vi "Process_old.vi"(8 "error in (no error)":errorcluster, 10 "DAQ Class.lvclass":refnum<class "DAQ Class.lvclass">, 11 "Intensity Processing in":refnum<class "Intensity Processing.lvclass">) -> (0 "error out":errorcluster, 3 "Intensity Processing out":refnum<class "Intensity Processing.lvclass">)   [LabVIEW 2014]
uses:
  <vilib>/Analysis/NI_AALPro.lvlib
  DAQ/DAQ Control Functional Global States.ctl
  <vilib>/Analysis/4window.llb/Hanning Window (DBL).vi
  <vilib>/Analysis/2dsp.llb/Real FFT.vi
  DAQ/DAQ Class.lvclass
  Processing.lvclass
  Intensity Processing.lvclass
panel:
  out "Log?":bool=TRUE
  out "Intensity Graph":sgl[][](graph)
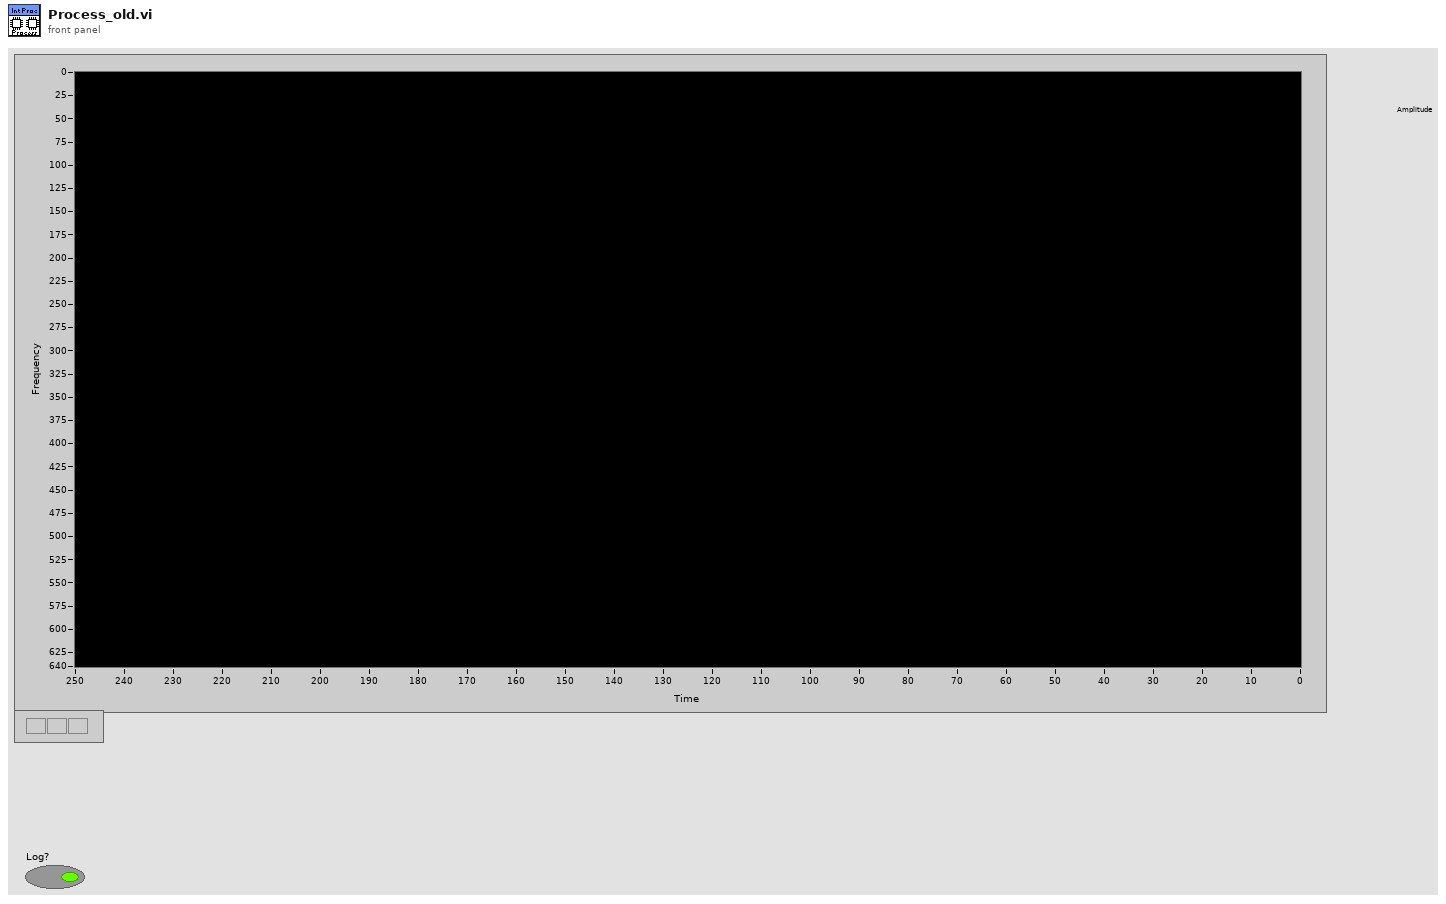
[diagram p1: front panel]
types:
  T1 = typedef "DAQ Class.lvclass/DAQ Parameters.ctl" = cluster{"Points Per A-Scan":u32, "A-Scans Per B-Scan":u32, "Number of B-Scans":u32, "A-Scans Per Transfer":u32, "Trigger Voltage":sgl, "Trigger Source":T2, "Trigger Slope":T3, "Channel":T4, "Clock":T5, "Bits per Sample":dbl, "Range":dbl}
  T2 = typedef "DAQ Class.lvclass/Trigger Source.ctl" = enum16{"External", "Channel A", "Channel B"}
  T3 = typedef "DAQ Class.lvclass/Trigger Slope.ctl" = enum16{"Rising", "Falling"}
  T4 = typedef "OCT DAQ Channel Data Type.ctl" = enum16{"Channel 1", "Channel 2", "Channel 1 and 2"}
  T5 = typedef "DAQ Class.lvclass/Clock Control.ctl" = enum16{"Internal Clock", "External Clock"}
  T6 = enum16{"open", "replace", "create", "open or create", "replace or create", "replace or create with confirmation"}
  T7 = typedef "DAQ Control Functional Global States.ctl" = enum16{"Status", "Set Processing Finished", "Reset", "Clear", "Set DAQ Finished"}
  T8 = typedef "LVCursorListTypeDef.ctl" = cluster{"Name":string, "Color":u32, "Style":u8, "Point Style":u8, "Name Visible":bool, "Allow Drag":bool, "Cursor Mode":u32, "Plot":i32, "Index":i32, "Position":cluster{"X":dbl, "Y":dbl}, "X Scale":u32, "Y Scale":u32, "Watch Plots":i32[], "Watch All Plots":bool, "Plot Area":i32, "Label Offset":cluster{"X":dbl, "Y":dbl}}[]
  T9 = cluster{"Name":string, "Color":u32, "Style":u8, "Point Style":u8, "Name Visible":bool, "Allow Drag":bool, "Cursor Mode":u32, "Plot":i32, "Index":i32, "Position":cluster{"X":dbl, "Y":dbl}, "X Scale":u32, "Y Scale":u32, "Watch Plots":i32[], "Watch All Plots":bool, "Plot Area":i32, "Label Offset":cluster{"X":dbl, "Y":dbl}}
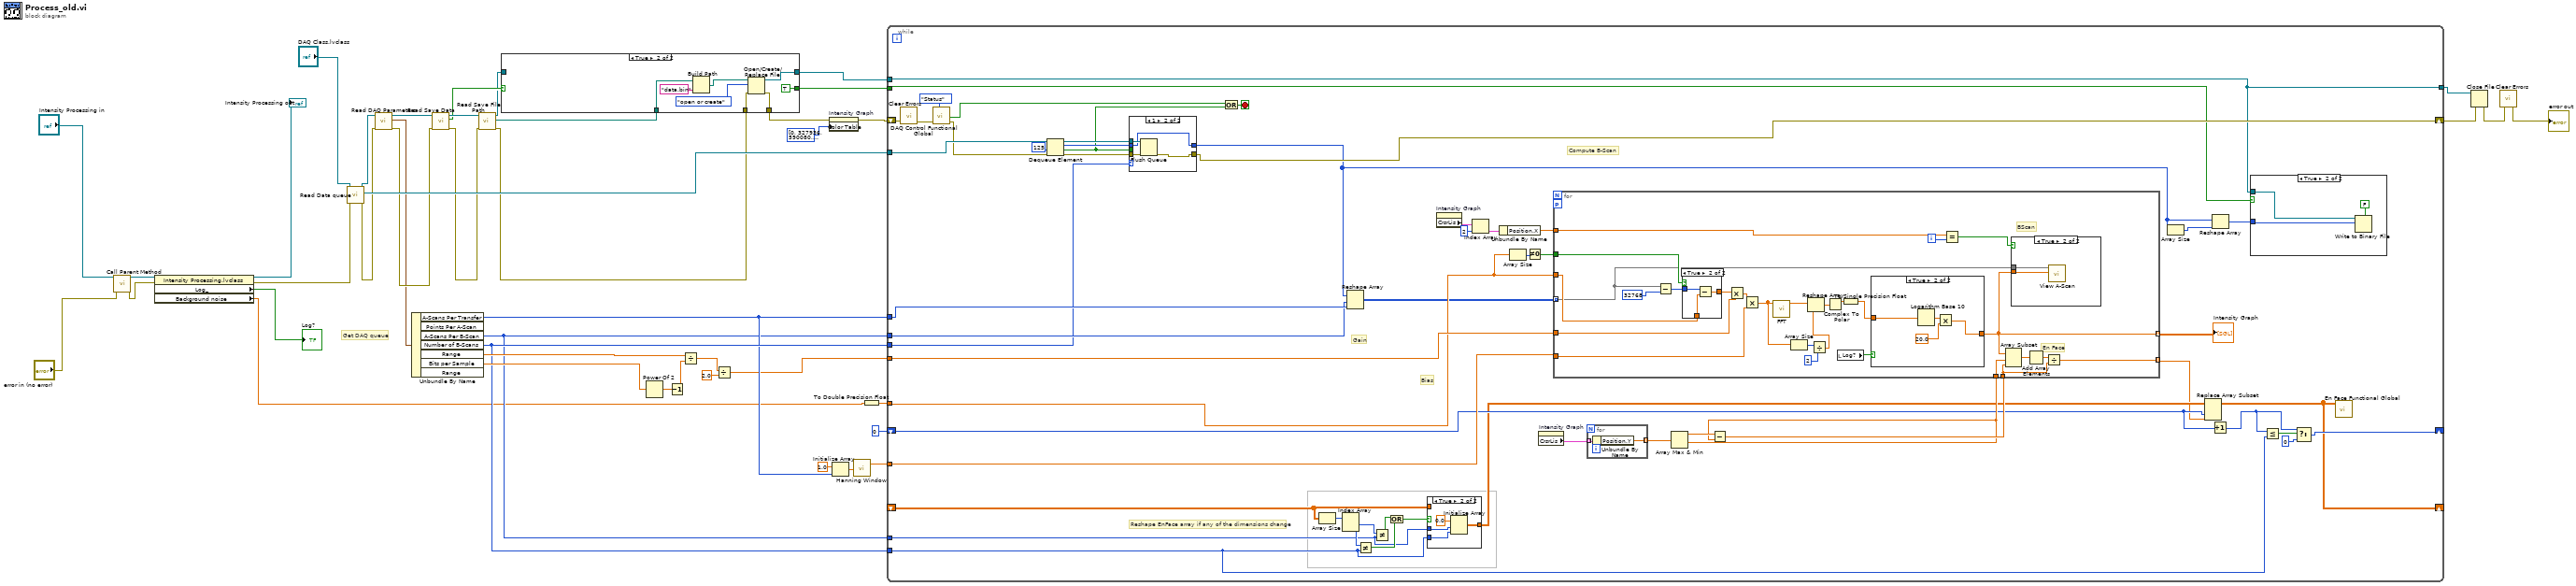
[diagram p0: block diagram]
diagram:
  # "Get DAQ queue"
  n1 = call-parent "Call Parent Method"("error in (no error)"="error in (no error)", "Processing in"="Intensity Processing in") -> ("error out"=w23:errorcluster, "Processing out"=w25:refnum<class "Intensity Processing.lvclass">)  [unwired: 8 in]
  n2 = property class="Intensity Processing.lvclass"(reference=w25, error in=w23) -> (reference out=→"Intensity Processing out":refnum<class "Intensity Processing.lvclass">, error out=w22:errorcluster, "Log_"=→"Log?":bool, "Background noise"=w3:dbl[])
  n3 = call-dynamic "Read Data queue.vi"("error in (no error)"=w22, "DAQ Class in"="DAQ Class.lvclass") -> ("error out"=w43:errorcluster, "Data queue"=w44:refnum<queue>, "DAQ Class out"=w42:refnum<class "DAQ Class.lvclass">)  [unwired: 7 in]
  n4 = call-dynamic "Read DAQ Parameters.vi"("error in (no error)"=w43, "DAQ Class in"=w42) -> ("error out"=w18:errorcluster, "DAQ Parameters"=w8:T1, "DAQ Class out"=w20:refnum<class "DAQ Class.lvclass">)  [unwired: 7 in]
  n5 = Unbundle By Name(w8) -> ("Points Per A-Scan"=w13:u32, "A-Scans Per B-Scan"=w12:u32, "Number of B-Scans"=w14:u32, "Range"=w39:dbl, "Bits per Sample"=w40:dbl)  [unwired: 2 out]
  n6 = call-dynamic "Read Save Data.vi"("error in (no error)"=w18, "DAQ Class in"=w20) -> ("error out"=w19:errorcluster, "Save Data"=w16:bool, "DAQ Class out"=w17:refnum<class "DAQ Class.lvclass">)  [unwired: 7 in]
  n7 = call-dynamic "Read Save File Path.vi"("error in (no error)"=w19, "DAQ Class in"=w17) -> ("error out"=w32:errorcluster, "Save File Path"=w15:path, "DAQ Class out"=w7:refnum<class "DAQ Class.lvclass">)  [unwired: 7 in]
  n8 = case shown="True" w16 {
    selector: w16 -> [w46 _]
    tunnel: w32 -> [w47 w55]
    tunnel: [w47 w54] -> w10
    tunnel: [_ w53] -> w36
    tunnel: [w46 TRUE] -> w35
    tunnel: w15 -> [_ w51]
    tunnel: w7 -> [_ _]
    frame False {
    }
    frame True {
      n9 = Build Path(base path=w51, name or relative path="data.bin") -> (appended path=w50:path)
      n10 = Open/Create/Replace File(file path (use dialog)=w50, error in=w55, operation (0:open)=T6."open or create") -> (refnum out=w53:refnum<file>, error out=w54:errorcluster)  [unwired: 3 in, 1 out]
    }
  }
  n11 = Power Of 2(x=w40) -> (2^x=w41:dbl)
  n12 = Decrement(x=w41) -> (x-1=w38:dbl)
  n13 = Divide(x=w39, y=w38) -> (x/y=w6:dbl)
  n14 = Divide(x=w6, y=2.0) -> (x/y=w5:dbl)
  n15 = property on="Intensity Graph" class="IntGraph (strict)"(error in=w10, "Color Table"=u32[] [0, 327936, 590080, 852224, 983296, 1114624, 1180160, 1311232, 1442304, 1573632, 1704704, 1770240, 1901312, 1966848, 2098176, 2163712, 2294784, 2491392, 2557184, 2688256, 2753792, 2884864, 2950656, 3081728, 3147264, 3344129, 3475457, 3540993, 3672321, 3738113, 3869185, 3934977, 4066305, 4197633, 4328961, 4394497, 4460289, 4591617, 4657409, 4788481, 4854273, 4985601, 5116929, 5248257, 5314049, 5379841, 5511169, 5576961, 5708033, 5773825, 5905153, 6036482, 6167810, 6233346, 6299138, 6430466, 6496258, 6562050, 6693634, 6759426, 6890754, 7022082, 7087874, 7153666, 7284994, 7350786, 7482114, 7547906, 7613698, 7745026, 7876354, 8007682, 8073474, 8139522, 8205314, 8336642, 8467970, 8533763, 8599555, 8665347, 8731139, 8862467, 8993795, 9059587, 9125380, 9191428, 9257220, 9388548, 9454340, 9520132, 9585924, 9717253, 9848837, 9914629, 9980165, 10045957, 10177541, 10243334, 10309126, 10375174, 10440966, 10572294, 10703623, 10769416, 10835208, 10901256, 10967049, 11033097, 11033609, 11099401, 11165450, 11231242, 11231754, 11297547, 11363339, 11429131, 11495180, 11495692, 11561740, 11693069, 11758861, 11759373, 11825165, 11891214, 11957006, 12022799, 12023311, 12089103, 12220944, 12286736, 12286736, 12352529, 12418577, 12484370, 12550162, 12615954, 12681747, 12747796, 12813588, 12813845, 12879894, 12945686, 13077015, 13142808, 13143064, 13208856, 13274905, 13340697, 13340953, 13472282, 13538075, 13604379, 13670172, 13735964, 13801757, 13867550, 13933343, 13999392, 13999648, 14065441, 14131234, 14197027, 14197541, 14263334, 14329383, 14395176, 14460969, 14592553, 14658346, 14724139, 14789932, 14790189, 14856238, 14922287, 14988080, 15053873, 15054130, 15119923, 15185972, 15251765, 15317559, 15383353, 15449146, 15449660, 15515454, 15515968, 15516226, 15582021, 15582278, 15582536, 15648587, 15648844, 15714639, 15714897, 15715155, 15780949, 15781463, 15847256, 15847770, 15848028, 15913823, 15914081, 15979875, 15980133, 15980391, 16046441, 16046444, 16046703, 16046705, 16112500, 16113015, 16113274, 16113277, 16179072, 16179330, 16179588, 16245384, 16245387, 16245389, 16245648, 16311443, 16376982, 16377241, 16377499, 16443294, 16443553, 16443555, 16443815, 16509866, 16510124, 16510127, 16575923, 16575924, 16576182, 16576441, 16576443, 16576702, 16576705, 16576963, 16577222, 16577224, 16577482, 16577485, 16577743, 16577745, 16578004, 16578262, 16578264, 16578523, 16578782, 16579040, 16579299, 16579301, 16579303, 16579562, 16579821]) -> (error out=w11:errorcluster)  [unwired: 1 in, 1 out]
  n16 = Initialize Array(1.0 ("element"), w13) -> (w2:dbl[])
  n17 = call-poly <vilib>:"Hanning Window.vi"("X"=w2) -> ("Windowed X"=w30:dbl[])  [unwired: 1 out]
  n18 = To Double Precision Float(number=w3) -> (double precision float=w4:dbl[])
  n19 = while {
    tunnel: w44 -> [w81]
    shift-right: [w75] -> w34
    shift-left: w11 -> [w108]
    tunnel: w5 -> [w79]
    tunnel: w13 -> [w87]
    tunnel: w12 -> [w86]
    tunnel: w30 -> [w109]
    tunnel: w36 -> [w66]
    tunnel: w35 -> [w65]
    tunnel: [w66] -> w33
    shift-right: [w96] -> _
    shift-left: _ -> [w95]
    shift-right: [w100] -> _
    shift-left: 0 -> [w101]
    tunnel: w12 -> [w88]
    tunnel: w14 -> [w78]
    tunnel: w14 -> [w64]
    tunnel: w4 -> [w68]
    stop <- w99 stop-if-true
    # "Compute B-Scan"
    # "Reshape EnFace array if any of the dimensions change"
    # "Bias"
    # "Gain"
    n20 = call <vilib>:"Clear Errors.vi"("error in (no error)"=w108) -> ("error out"=w107:errorcluster)  [unwired: 5 in, 1 out]
    n21 = call "DAQ Control Functional Global.vi"("State"=DAQ_Control_Functional_Global_States."Status", "Error In"=w107) -> ("Error Out"=w80:errorcluster, "Reset?"=w82:bool)  [unwired: 6 in, 2 out]
    n22 = Dequeue Element(queue=w81, timeout in ms (-1)=125, error in (no error)=w80) -> (queue out=w71:refnum<queue>, element=w72:u16[], timed out?=w63:bool, error out=w70:errorcluster)
    n23 = case shown="1" w64 {
      tunnel: w72 -> [w114 w115]
      tunnel: w71 -> [_ w117]
      tunnel: [w114 w115] -> w57
      tunnel: w63 -> [_ _]
      tunnel: w70 -> [w113 w118]
      tunnel: [w113 w116] -> w75
      frame 0, Default {
      }
      frame 1 {
        n24 = Flush Queue(queue=w117, error in (no error)=w118) -> (error out=w116:errorcluster)  [unwired: 2 out]
      }
    }
    n25 = Or(x=w82, y=w63) -> (x .or. y?=w99:bool)
    n26 = Array Size(array=w95) -> (size(s)=w94:i32[])
    n27 = Index Array(array=w94) -> (element #1=w92:i32, element #2=w93:i32)  [unwired: 2 in]
    n28 = Reshape Array(w57, w86, w87) -> (w58:u16[][])
    n29 = Not Equal?(x=w93, y=w78) -> (x != y?=w90:bool)
    n30 = Not Equal?(x=w92, y=w88) -> (x != y?=w89:bool)
    n31 = Or(x=w89, y=w90) -> (x .or. y?=w91:bool)
    n32 = case shown="True" w91 {
      tunnel: w88 -> [_ w160]
      tunnel: w78 -> [_ w159]
      tunnel: [w157 w158] -> w97
      tunnel: w95 -> [w157 _]
      frame False {
      }
      frame True {
        n33 = Initialize Array(sgl 0.0 ("element"), w160, w159) -> (w158:sgl[][])
      }
    }
    n34 = property on="Intensity Graph" class="IntGraph (strict)"() -> ("CrsrLis"=w62:T8)  [unwired: 2 in, 2 out]
    n35 = Index Array(array=w62, index=2) -> (element=w60:T9)
    n36 = Unbundle By Name(w60) -> ("Position.X"=w59:dbl)
    n37 = Array Size(array=w68) -> (size(s)=w77:i32)
    n38 = Not Equal To 0?(x=w77) -> (x != 0?=w76:bool)
    n39 = property on="Intensity Graph" class="IntGraph (strict)"() -> ("CrsrLis"=w103:T8)  [unwired: 2 in, 2 out]
    n40 = for {
      tunnel: w103 -> [w163] mode=indexing
      tunnel: [w162] -> w102 mode=indexing
      n41 = Unbundle By Name(w163) -> ("Position.Y"=w162:dbl)
    }
    n42 = Array Max & Min(array=w102) -> (max value=w106:dbl, min value=w104:dbl)  [unwired: 2 out]
    n43 = Subtract(x=w106, y=w104) -> (x-y=w105:dbl)
    n44 = for {
      tunnel: w109 -> [w145]
      tunnel: [w120] -> w69 mode=indexing
      tunnel: w105 -> [w140]
      tunnel: w104 -> [w143]
      tunnel: [w119] -> w74 mode=indexing
      tunnel: w79 -> [w138]
      tunnel: w58 -> [w124] mode=indexing
      tunnel: w68 -> [w130]
      tunnel: w76 -> [w128]
      workers-P: _ -> [_]
      tunnel: w59 -> [w126]
      i -> [w127]
      # "BScan"
      # "En Face"
      n45 = Subtract(x=w124, y=32768) -> (x-y=w131:i32[])
      n46 = case shown="True" w128 {
        tunnel: w131 -> [w148 w151]
        tunnel: w130 -> [_ w150]
        tunnel: [w148 w149] -> w129
        frame False {
        }
        frame True {
          n47 = Subtract(x=w151, y=w150) -> (x-y=w149:dbl[])
        }
      }
      n48 = Multiply(x=w129, y=w138) -> (x*y=w132:dbl[])
      n49 = Multiply(x=w132, y=w145) -> (x*y=w134:dbl[])
      n50 = call-poly <vilib>:"FFT.vi"("X"=w134) -> ("FFT {X}"=w144:cdb[])  [unwired: 9 in, 1 out]
      n51 = Array Size(array=w134) -> (size(s)=w137:i32)
      n52 = Divide(x=w137, y=2) -> (x/y=w135:dbl)
      n53 = Reshape Array(w144, w135) -> (w123:cdb[])
      n54 = Complex To Polar(r * e^(i*theta)=w123) -> (r=w122:dbl[])  [unwired: 1 out]
      n55 = local read "Log?"() -> (w139:bool)
      n56 = To Single Precision Float(number=w122) -> (single precision float=w121:sgl[])
      n57 = case shown="True" w139 {
        tunnel: w121 -> [w152 w156]
        tunnel: [w152 w153] -> w120
        frame False {
        }
        frame True {
          n58 = Logarithm Base 10(1:w156) -> (0:w155:sgl[])
          n59 = Multiply(x=w155, y=sgl 20.0 ("element")) -> (x*y=w153:sgl[])
        }
      }
      n60 = Equal?(x=w126, y=w127) -> (x = y?=w125:bool)
      n61 = Array Subset(array=w120, index=w143, length=w140) -> (w142:sgl[])
      n62 = case shown="True" w125 {
        tunnel: w124 -> [_ w147]
        tunnel: w120 -> [_ w146]
        frame False {
        }
        frame True {
          n63 = call "View A-Scan.vi"("A-Scan Processed"=w146, "A-Scan (Raw)"=w147) -> ()  [unwired: 10 in]
        }
      }
      n64 = Add Array Elements(numeric array=w142) -> (sum=w141:sgl)
      n65 = Divide(x=w141, y=w140) -> (x/y=w119:dbl)
    }
    "Intensity Graph" <- w69
    n66 = Array Size(array=w57) -> (size(s)=w56:i32)
    n67 = Replace Array Subset(array=w97, new element=w74, index (col)=w101) -> (w96:sgl[][])  [unwired: 1 in]
    n68 = Increment(x=w101) -> (x+1=w84:i32)
    n69 = Reshape Array(w57, w56) -> (w67:u16[])
    n70 = case shown="True" w65 {
      tunnel: w66 -> [_ w111]
      tunnel: w67 -> [_ w110]
      frame False {
      }
      frame True {
        n71 = Write to Binary File(file (use dialog)=w111, data=w110, 5:FALSE ("prepend array or string size? (T)")) -> ()  [unwired: 3 in, 3 out]
      }
    }
    n72 = Less Or Equal?(x=w84, y=w78) -> (x <= y?=w85:bool)
    n73 = Select(t=w84, s=w85, f=0) -> (s? t:f=w100:i32)
    n74 = call "En Face Functional Global.vi"("Input"=w96) -> ()  [unwired: 9 in, 2 out]
  }
  n75 = Close File(refnum=w33, error in=w34) -> (error out=w28:errorcluster)  [unwired: 1 out]
  n76 = call <vilib>:"Clear Errors.vi"("error in (no error)"=w28) -> ("error out"=→"error out":errorcluster)  [unwired: 5 in, 1 out]
